vi "App - analyze RUS V6.vi"() -> ()   [LabVIEW 2018] (continued)
              tunnel: w1145 -> [w1161]
              tunnel: w1144 -> [w1159]
              frame #0 {
                n513 = call "cursor window logic V2.vi"("CursIdx"=w1151, "cursor window action"=cursor_window_action."cursor moves", "cursor window in"=w1152) -> ("cursor window out"=w1149:refnum<vi>)  [unwired: 7 in, 1 out]
                n514 = call "single fit V5.vi"("find fit action"=find_peak_action."fragment window moves", "cursor bracket: fragment  ref"=w1149) -> ("single fit parameters out"=w1154:T21, "omega map parameters out"=w1155:T22, "lorentzian out"=w1153:T11)  [unwired: 9 in, 2 out]
                n515 = local write "parameters: center detection"(w1154) -> ()
                n516 = local write "parameters: omega map"(w1155) -> ()
                n517 = local write "lorentzian"(w1153) -> ()
                n518 = Unbundle By Name(w1153) -> ("f (Hz)"=w1157:dbl)
              }
              frame #1 {
                w1160 = enum16{"", "read", "write"}."write"  # action
                w1162 = "update freq/atten"  # t.folder
                n519 = call "replace cursor - plot ref.vi"("action"=w1160, "cursor index"=9, "new X"=w1159, "Plot ref in"=w1161) -> ()  [unwired: 5 in, 3 out]
                n520 = Generate User Event(user event=w1163, event data cluster=w1162) -> ()  [unwired: 2 in, 2 out]
              }
            }
          }
          frame 3 {
            # "blue cursor"
            # "cusor 0 in \"complex plane\", \"geometry \" and l\"inear map \" is tied to cursor in \"fragment\" window"
            n521 = Unbundle By Name(w1166) -> ("normalized z"=w1193:cdb[], "omega in window"=w1192:dbl[], "inverse"=w1169:cdb[], "linear"=w1170:cdb[], "omega around"=w1171:dbl[])
            n522 = call "replace cursor - plot ref.vi"("action"=enum16{"", "read", "write"}."read", "cursor index"=w1189, "Plot ref in"=w1165) -> ("read X"=w1190:dbl)  [unwired: 6 in, 2 out]
            n523 = Threshold 1D Array(2:w1190, 3:w1192) -> (0:w1183:dbl)  [unwired: 1 in]
            n524 = Threshold 1D Array(2:w1190, 3:w1171) -> (0:w1173:dbl)  [unwired: 1 in]
            n525 = Index Array(array=w1193, index=w1183) -> (element=w1188:cdb)
            n526 = Index Array(array=w1170, index=w1173) -> (element=w1175:cdb)
            n527 = Index Array(array=w1171, index=w1173) -> (element=w1172:dbl)
            n528 = Index Array(array=w1169, index=w1173) -> (element=w1182:cdb)
            n529 = Complex To Re/Im(x + iy=w1175) -> (x=w1174:dbl)  [unwired: 1 out]
            n530 = Complex To Re/Im(x + iy=w1182) -> (x=w1179:dbl, y=w1178:dbl)
            n531 = control-ref of="Plot: linear map"() -> (w1168:refnum<vi>)
            n532 = Complex To Re/Im(x + iy=w1188) -> (x=w1187:dbl, y=w1186:dbl)
            n533 = control-ref of="Plot: geometry"() -> (w1167:refnum<vi>)
            n534 = call "replace cursor - plot ref.vi"("action"=enum16{"", "read", "write"}."write" ("Enum"), "cursor index"=0, "new  Y"=w1186, "new X"=w1187, "Plot ref in"=w1164) -> ()  [unwired: 4 in, 3 out]
            n535 = call "replace cursor - plot ref.vi"("action"=enum16{"", "read", "write"}."write" ("Enum"), "cursor index"=0, "new  Y"=w1174, "new X"=w1172, "Plot ref in"=w1168) -> ()  [unwired: 4 in, 3 out]
            n536 = call "replace cursor - plot ref.vi"("action"=enum16{"", "read", "write"}."write" ("Enum"), "cursor index"=0, "new  Y"=w1178, "new X"=w1179, "Plot ref in"=w1167) -> ()  [unwired: 4 in, 3 out]
          }
        }
      }
      event "Plot: Time": Cursor Release {
        w1200 = enum16{"hide", "show x", "show y", "show (x,y)"}."hide"  # label
        w1201 = enum16{"", "read", "write"}."write"  # action
        w1202 = "same"  # next temperature
        n537 = event-data() -> ("CursIdx"=w1198:i32)  [unwired: 1 in]
        n538 = call "replace cursor - plot ref.vi"("label"=w1200, "action"=w1201, "cursor index"=w1198, "Plot ref in"=w1199) -> ()  [unwired: 5 in, 3 out]
        n539 = Generate User Event(user event=w1203, event data cluster=w1202) -> ()  [unwired: 2 in, 2 out]
        n540 = call "slide controller.vi"("slide action"=slide_action."stop slide", "slide control"=w1195) -> ()  [unwired: 6 in, 4 out]
        n541 = call "follow the peak controller.vi"("action"=follow_the_peak_action."make dirty", "follow the peak ref"=w1197) -> ()  [unwired: 8 in, 2 out]
      }
      event Key Down {
        n542 = event-data() -> ("Type"=w1208:T20, "Char"=w1223:i16, "VKey"=w1212:T19)  [unwired: 1 in]
        "Char" <- w1223
        "VKey" <- w1212
        "Type" <- w1208
        n543 = case shown="\"ASCII\", Default" w1212 {
          selector: w1212 -> [_ _ _ _ _ _ _ _ _ _ _ _ w1395 _ _ _ _ _ _ _ _ _ _ _ _ _ _ _ _ _ _ _ _ _ _ _ _ _ _ _ _ _ _ _ _ _ _ _ _ _]
          tunnel: w1223 -> [w1242 _ _ _ _ _ _ _ _ _ _ _ _ _ _ _ _ _ _ _ _ _ _ _ _ _ _ _ _ _ _ _ _ _ _ _ _ _ _ _ _ _ _ _ _ _ _ _ _ _]
          tunnel: w1222 -> [w1241 _ _ _ _ _ _ _ _ _ _ _ _ _ _ _ _ _ _ _ _ _ _ _ _ _ _ _ _ _ _ _ _ _ _ _ _ _ _ _ _ _ _ _ _ _ _ _ _ _]
          tunnel: w1221 -> [w1240 _ _ _ _ _ _ _ _ _ _ _ _ _ _ _ _ _ _ _ _ _ _ _ _ _ _ _ _ _ _ _ _ _ _ _ _ _ _ _ _ _ _ _ _ _ _ _ _ _]
          tunnel: w1220 -> [w1239 _ _ _ _ _ _ _ _ _ _ _ _ _ _ _ _ _ _ _ _ _ _ _ _ _ _ _ _ _ _ _ _ _ _ _ _ _ _ _ _ _ _ _ _ _ _ _ _ _]
          tunnel: w1219 -> [w1238 _ _ _ _ _ _ _ _ _ _ _ _ _ _ _ _ _ _ _ _ _ _ _ _ _ _ _ _ _ _ _ _ _ _ _ _ _ _ _ _ _ _ _ _ _ _ _ _ _]
          tunnel: w1218 -> [w1237 _ _ _ _ _ _ _ _ _ _ _ w1390 _ _ _ _ _ _ _ _ _ _ _ _ _ _ _ _ _ _ _ _ _ _ _ _ _ _ _ _ _ _ _ _ _ _ _ _ _]
          tunnel: w1217 -> [w1236 _ _ _ _ _ _ _ _ _ _ _ _ _ _ _ _ _ _ _ _ _ _ _ _ _ _ _ _ _ _ _ _ _ _ _ _ _ _ _ _ _ _ _ _ _ _ _ _ _]
          tunnel: w1216 -> [w1235 _ _ _ _ _ _ _ _ _ _ _ _ _ _ _ _ _ _ _ _ _ _ _ _ _ _ _ _ _ _ _ _ _ _ _ _ _ _ _ _ _ _ _ _ _ _ _ _ _]
          tunnel: w1215 -> [w1234 _ _ _ _ _ _ _ _ _ _ _ _ _ _ _ _ _ _ _ _ _ _ _ _ _ _ _ _ _ _ _ _ _ _ _ _ _ _ _ _ _ _ _ _ _ _ _ _ _]
          tunnel: w1214 -> [w1233 _ _ _ _ _ _ _ _ _ _ _ w1391 _ _ _ _ _ _ _ _ _ _ _ _ _ _ _ _ _ _ _ _ _ _ _ _ _ _ _ _ _ _ _ _ _ _ _ _ _]
          tunnel: w1213 -> [w1232 _ _ _ _ _ _ _ _ _ _ _ w1394 _ _ _ _ _ _ _ _ _ _ _ _ _ _ _ _ _ _ _ _ _ _ _ _ _ _ _ _ _ _ _ _ _ _ _ _ _]
          tunnel: w1211 -> [w1230 _ _ _ _ _ _ _ _ _ _ _ w1392 _ _ _ _ _ _ _ _ _ _ _ _ _ _ _ _ _ _ _ _ _ _ _ _ _ _ _ _ _ _ _ _ _ _ _ _ _]
          tunnel: w1210 -> [w1231 _ w1383 _ _ _ _ _ _ _ _ _ _ _ _ _ _ _ _ _ _ _ _ _ _ _ _ _ _ _ _ _ _ _ _ _ _ _ _ _ _ _ _ _ _ _ _ _ _ _]
          tunnel: w1209 -> [_ _ w1384 _ _ _ _ _ _ _ _ _ _ _ _ _ _ _ _ _ _ _ _ _ _ _ _ _ _ _ _ _ _ _ _ _ _ _ _ _ _ _ _ _ _ _ _ _ _ _]
          tunnel: w1208 -> [_ _ _ _ _ _ _ _ _ _ _ _ _ _ _ _ _ _ _ _ _ _ _ _ _ _ _ _ _ _ _ _ _ _ _ _ _ _ _ _ _ _ _ _ _ _ _ _ _ _]
          tunnel: w1207 -> [w1227 _ _ _ _ _ _ _ _ _ _ _ _ _ _ _ _ _ _ _ _ _ _ _ _ _ _ _ _ _ _ _ _ _ _ _ _ _ _ _ _ _ _ _ _ _ _ _ _ _]
          tunnel: w1206 -> [w1226 _ _ _ _ _ _ _ _ _ _ _ _ _ _ _ _ _ _ _ _ _ _ _ _ _ _ _ _ _ _ _ _ _ _ _ _ _ _ _ _ _ _ _ _ _ _ _ _ _]
          tunnel: w1205 -> [w1225 _ _ _ _ _ _ _ _ _ _ _ _ _ _ _ _ _ _ _ _ _ _ _ _ _ _ _ _ _ _ _ _ _ _ _ _ _ _ _ _ _ _ _ _ _ _ _ _ _]
          tunnel: w1204 -> [w1224 _ w1380 _ _ _ _ _ _ _ _ _ _ _ _ _ _ _ _ _ _ _ _ _ _ _ _ _ _ _ _ _ _ _ _ _ _ _ _ _ _ _ _ _ _ _ _ _ _ _]
          frame "ASCII", Default {
            # "[  - next temperature -- Down\n]  - next temperature -- Up\n\" \" - recalculate , stop sliding\n>  - start slide Up\n< -  start slide Down\n\netc..."
            n544 = case shown="111" w1242 {
              tunnel: w1241 -> [_ w1254 w1258 _ _ _ _ w1278 w1284 _ _ _ _ _ _ _ _ _ _ _ _ _ _ _ _ _ _ _ _ _ _ _ _]
              tunnel: TRUE -> [_ _ _ _ _ _ _ _ _ _ _ _ _ _ _ _ _ _ _ _ _ _ _ _ _ _ _ _ _ _ _ w1375 _]
              tunnel: w1239 -> [_ _ _ _ _ _ _ _ _ _ _ _ _ _ _ _ _ _ _ _ _ _ _ _ _ _ _ _ _ _ _ _ _]
              tunnel: FALSE -> [_ _ _ _ _ _ _ _ _ _ _ _ _ _ _ _ _ _ _ _ _ _ _ _ _ _ _ _ _ _ _ w1376 _]
              tunnel: w1240 -> [_ _ _ _ _ _ _ _ _ _ _ _ _ _ _ _ _ _ _ _ w1328 _ w1342 _ _ _ _ _ _ _ _ _ _]
              tunnel: w1238 -> [_ _ _ _ _ _ _ _ _ _ _ _ _ _ _ _ _ _ _ _ _ w1340 _ _ _ _ _ _ _ _ _ _ _]
              tunnel: w1237 -> [_ _ _ w1263 _ _ _ _ _ _ _ _ _ _ _ _ _ _ _ _ _ _ _ _ _ _ _ _ _ _ _ w1379 _]
              tunnel: w1236 -> [w1247 _ _ w1260 w1264 w1267 w1271 _ _ _ _ _ _ _ w1305 _ _ _ w1313 _ w1329 _ _ w1348 w1359 w1360 w1362 _ _ _ w1372 _ _]
              tunnel: w1235 -> [_ _ _ _ _ _ _ _ _ _ _ _ _ _ _ _ _ _ _ _ _ _ _ _ _ _ _ _ _ _ _ _ _]
              tunnel: w1234 -> [_ _ _ _ _ _ _ _ _ _ _ _ _ w1302 _ _ _ _ _ _ _ _ _ _ _ _ _ _ _ _ _ _ _]
              tunnel: w1233 -> [_ _ _ _ _ _ _ _ _ _ _ _ w1293 _ _ _ _ _ _ _ _ _ _ _ _ _ _ _ _ _ _ _ _]
              tunnel: w1232 -> [w1249 _ _ _ _ _ _ _ _ _ w1287 w1289 _ _ _ _ _ _ _ w1315 _ _ _ _ _ _ _ w1366 w1368 w1370 _ _ _]
              tunnel: w1231 -> [_ _ _ _ _ _ _ _ _ _ _ _ _ _ _ _ _ _ _ w1318 _ _ _ _ _ _ _ _ _ _ _ _ _]
              tunnel: w1230 -> [_ _ _ _ _ _ _ _ _ w1285 _ _ _ _ _ _ _ _ _ w1319 _ _ _ _ _ _ _ _ _ _ _ _ _]
              tunnel: w1227 -> [_ _ _ _ _ _ _ _ _ _ _ _ _ _ _ _ _ _ _ _ _ _ _ _ _ _ _ _ _ _ _ _ _]
              tunnel: w1226 -> [w1246 _ _ _ _ _ _ _ _ _ _ _ _ _ _ w1307 w1310 _ _ _ _ _ _ _ _ _ _ _ _ _ _ _ _]
              tunnel: w1225 -> [w1243 w1252 w1255 _ _ _ _ w1273 w1281 _ _ _ _ _ _ _ _ _ _ _ _ _ _ _ _ _ _ _ _ _ _ _ _]
              tunnel: w1224 -> [_ _ _ _ _ _ _ _ _ _ _ _ _ _ w1303 _ _ _ _ _ _ _ _ w1343 w1356 _ _ _ _ _ _ _ _]
              frame 32 {
                w1248 = "update delta freq"  # t.folder
                # "stop slide and/or recalculate"
                # "\"<space>\""
                # "recalculate"
                n545 = Generate User Event(user event=w1249, event data cluster="calc:peak" ("event data")) -> ()  [unwired: 2 in, 2 out]
                n546 = call "follow the peak controller.vi"("action"=follow_the_peak_action."make dirty", "follow the peak ref"=w1246) -> ()  [unwired: 8 in, 2 out]
                n547 = call "slide controller.vi"("slide action"=slide_action."stop slide", "slide control"=w1243) -> ()  [unwired: 6 in, 4 out]
                n548 = Generate User Event(user event=w1247, event data cluster=w1248) -> ()  [unwired: 2 in, 2 out]
              }
              frame 44 {
                w1253 = "next"  # event data
                # "slide down"
                # "\" <\""
                n549 = Generate User Event(user event=w1254, event data cluster=w1253) -> ()  [unwired: 2 in, 2 out]
                n550 = call "slide controller.vi"("slide action"=slide_action."slide DOWN", "slide control"=w1252) -> ()  [unwired: 6 in, 4 out]
              }
              frame 46 {
                w1257 = "next"  # event data
                # "slide up"
                # ">"
                n551 = Generate User Event(user event=w1258, event data cluster=w1257) -> ()  [unwired: 2 in, 2 out]
                n552 = call "slide controller.vi"("slide action"=slide_action."slide UP", "slide control"=w1255) -> ()  [unwired: 6 in, 4 out]
              }
              frame 47 {
                w1261 = "update delta freq"  # t.folder
                (unwired) FALSE ("event data")
                # "\"/\""
                n553 = Generate User Event(user event=w1263, event data cluster="scale:frequency window" ("event data")) -> (error out=w1259:errorcluster)  [unwired: 2 in, 1 out]
                n554 = Generate User Event(user event=w1260, event data cluster=w1261, error in=w1259) -> ()  [unwired: 1 in, 2 out]
              }
              frame 59 {
                w1265 = "next peak"  # event data
                n555 = Generate User Event(user event=w1264, event data cluster=w1265) -> ()  [unwired: 2 in, 2 out]
              }
              frame 39 {
                n556 = for {
                  tunnel: w1267 -> [w1270]
                  tunnel: string[] ["write freq file", "increment peak index", "clear freq points", "follow the peak -- init", "set time to left", "read freq file"] -> [w1268] mode=indexing
                  n557 = Wait (ms)(milliseconds to wait=u32 1000) -> ()  [unwired: 1 out]
                  n558 = Generate User Event(user event=w1270, event data cluster=w1268) -> ()  [unwired: 2 in, 2 out]
                  "script event" <- w1268
                }
              }
              frame 58 {
                w1272 = "increment peak index"  # event data
                n559 = Generate User Event(user event=w1271, event data cluster=w1272) -> ()  [unwired: 2 in, 2 out]
              }
              frame 60 {
                w1277 = "next"  # next temperature
                # "next DOWN"
                # "shift <"
                # "send \"next temperature"
                # "next temperature  -- Down"
                n560 = Generate User Event(user event=w1278, event data cluster=w1277) -> ()  [unwired: 2 in, 2 out]
                n561 = call "slide controller.vi"("slide action"=slide_action."slide DOWN", "slide control"=w1273) -> ("slide control OUT"=w1274:refnum<vi>)  [unwired: 6 in, 3 out]
                n562 = call "slide controller.vi"("slide action"=slide_action."stop slide", "slide control"=w1274) -> ()  [unwired: 6 in, 4 out]
              }
              frame 62 {
                w1283 = "next"  # next temperature
                (unwired) TRUE
                (unwired) -1
                (unwired) 1
                # "next UP"
                # "shift >"
                # "Up"
                # "send next temperature"
                n563 = Generate User Event(user event=w1284, event data cluster=w1283) -> ()  [unwired: 2 in, 2 out]
                n564 = call "slide controller.vi"("slide action"=slide_action."slide UP", "slide control"=w1281) -> ("slide control OUT"=w1280:refnum<vi>)  [unwired: 6 in, 3 out]
                n565 = call "slide controller.vi"("slide action"=slide_action."stop slide", "slide control"=w1280) -> ()  [unwired: 6 in, 4 out]
              }
              frame 63 {
                n566 = call "cursor window logic V2.vi"("cursor window action"=cursor_window_action."zoom X", "cursor window in"=w1285) -> ()  [unwired: 8 in, 2 out]
              }
              frame 92 {
                w1288 = "jump to a PID peak"  # calculate
                # "\"\\\""
                n567 = Generate User Event(user event=w1287, event data cluster=w1288) -> ()  [unwired: 2 in, 2 out]
              }
              frame 43 {
                w1290 = "overwrite peak PID"  # calculate
                # "\"\\\""
                n568 = Generate User Event(user event=w1289, event data cluster=w1290) -> ()  [unwired: 2 in, 2 out]
              }
              frame 97 {
                # "\"a\""
                # "all plot autoscale"
                # "\"a\""
                n569 = local read "all:max omega"() -> (w1299:dbl)
                n570 = local read "all:min omega"() -> (w1298:dbl)
                n571 = Add(x=w1299, y=w1298) -> (x+y=w1300:dbl)
                n572 = Subtract(x=w1299, y=w1298) -> (x-y=w1297:dbl)
                n573 = Divide(x=w1300, y=2.0) -> (x/y=w1294:dbl)
                n574 = Divide(x=w1297, y=1.5) -> (x/y=w1291:dbl)
                n575 = property on="Plot: All" class="XYGraph (strict)"("XScale.Maximum"=w1299, "XScale.Minimum"=w1298) -> ()  [unwired: 2 in, 2 out]
                n576 = call "cursor window logic V2.vi"("cursor window action"=cursor_window_action."change cen&win", "window"=w1291, "center"=w1294, "cursor window in"=w1293) -> ()  [unwired: 6 in, 2 out]
              }
              frame 99 {
                (unwired) 0.0 ("event data")
                # "show cursors"
                # "\"c\""
                n577 = Generate User Event(user event=w1302, event data cluster="cursors:check all" ("event data")) -> ()  [unwired: 2 in, 2 out]
              }
              frame 101 {
                w1306 = "clear freq points"  # t.folder
                # "erase freq points \n\nshortcut \"e\""
                n578 = Generate User Event(user event=w1305, event data cluster=w1306) -> ()  [unwired: 2 in, 2 out]
                n579 = call "freq file read-write controller.vi"("action"=save-read_action."erase event", "save/read"=w1303) -> ()  [unwired: 7 in, 3 out]
              }
              frame 102 {
                # "\"f\""
                n580 = call "follow the peak controller.vi"("action"=follow_the_peak_action."toggle omega", "follow the peak ref"=w1307) -> ()  [unwired: 8 in, 2 out]
              }
              frame 103 {
                n581 = call "follow the peak controller.vi"("action"=follow_the_peak_action."toggle gamma", "follow the peak ref"=w1310) -> ()  [unwired: 8 in, 2 out]
              }
              frame 104 {
                # "help  \"h\""
                n582 = local read "help toggle"() -> (w1312:bool)
                n583 = Not(x=w1312) -> (.not. x?=w1311:bool)
                n584 = local write "help toggle"(w1311) -> ()
                n585 = Control Help Window(1:w1311) -> ()  [unwired: 1 in]
              }
              frame 106 {
                # "j"
                n586 = Generate User Event(user event=w1313, event data cluster="set time to left" ("event data")) -> ()  [unwired: 2 in, 2 out]
              }
              frame 109 {
                # "\"m\""
                n587 = Unbundle By Name(w1318) -> ("f (Hz)"=w1316:dbl)
                n588 = call "Q - not nan and not zero.vi"("Numeric"=w1316) -> ("Boolean"=w1317:bool)  [unwired: 10 in]
                n589 = case shown="True" w1317 {
                  tunnel: w1319 -> [_ w1322]
                  tunnel: w1316 -> [_ w1321]
                  tunnel: w1315 -> [_ w1320]
                  frame False {
                  }
                  frame True {
                    n590 = flat-sequence {
                      tunnel: w1322 -> [w1325]
                      tunnel: w1321 -> [w1324]
                      tunnel: w1320 -> [w1326]
                      frame #0 {
                        n591 = call "cursor window logic V2.vi"("cursor window action"=cursor_window_action."check", "center"=w1324, "cursor window in"=w1325) -> ()  [unwired: 7 in, 2 out]
                      }
                      frame #1 {
                        w1327 = "calc:new cursor bracket"  # event data
                        n592 = Generate User Event(user event=w1326, event data cluster=w1327) -> ()  [unwired: 2 in, 2 out]
                      }
                    }
                  }
                }
              }
              frame 111 {
                # "\"o\""
                n593 = flat-sequence {
                  tunnel: w1329 -> [w1332]
                  tunnel: [w1331] -> w1330
                  tunnel: [w1334] -> _
                  tunnel: w1330 -> [w1335]
                  tunnel: w1328 -> [w1336]
                  frame #0 {
                    w1333 = "new temperature folder"  # t.folder
                    n594 = Generate User Event(user event=w1332, event data cluster=w1333) -> (error out=w1331:errorcluster)  [unwired: 2 in, 1 out]
                  }
                  frame #1 {
                    n595 = Generate User Event(user event=w1336, event data cluster="redraw:time", error in=w1335) -> (error out=w1334:errorcluster)  [unwired: 1 in, 1 out]
                  }
                }
              }
              frame 112 {
                # "\"p\""
                n596 = local read "show all pallets (p)"() -> (w1339:bool)
                n597 = Not(x=w1339) -> (.not. x?=w1338:bool)
                n598 = local write "show all pallets (p)"(w1338) -> ()
                n599 = Generate User Event(user event=w1340, event data cluster=w1338) -> ()  [unwired: 2 in, 2 out]
              }
              frame 113 {
                w1341 = "plot filter progress"  # event data
                # "q"
                n600 = Generate User Event(user event=w1342, event data cluster=w1341) -> ()  [unwired: 2 in, 2 out]
              }
              frame 114 {
                w1350 = "update delta freq"  # t.folder
                w1351 = "read freq file"  # t.folder
                # "make something to protect  from overwriting a file"
                # "\"r\""
                n601 = case shown="True" FALSE {
                  tunnel: w1348 -> [w1352 w1354]
                  tunnel: [w1352 w1353] -> w1347
                  frame False {
                  }
                  frame True {
                    w1355 = "clear freq points"  # t.folder
                    n602 = Generate User Event(user event=w1354, event data cluster=w1355) -> (user event out=w1353:refnum<user-event>)  [unwired: 2 in, 1 out]
                  }
                }
                n603 = call "freq file read-write controller.vi"("action"=save-read_action."read event", "save/read"=w1343) -> ()  [unwired: 7 in, 3 out]
                n604 = Generate User Event(user event=w1347, event data cluster=w1351) -> (user event out=w1349:refnum<user-event>, error out=w1346:errorcluster)  [unwired: 2 in]
                n605 = Generate User Event(user event=w1349, event data cluster=w1350, error in=w1346) -> ()  [unwired: 1 in, 2 out]
              }
              frame 115 {
                w1358 = "write freq file"  # t.folder
                # "\"s\""
                n606 = call "freq file read-write controller.vi"("action"=save-read_action."save event", "save/read"=w1356) -> ()  [unwired: 7 in, 3 out]
                n607 = Generate User Event(user event=w1359, event data cluster=w1358) -> ()  [unwired: 2 in, 2 out]
              }
              frame 116 {
                w1361 = "lookup read from list"  # t.folder
                # "\"t\""
                n608 = Generate User Event(user event=w1360, event data cluster=w1361) -> ()  [unwired: 2 in, 2 out]
              }
              frame 117 {
                w1363 = "latest temperature"  # t.folder
                n609 = disable-structure shown="Disabled" {
                  disable-tunnel: w1362 -> [w1364 _]
                  frame Disabled {
                    w1365 = "append frequency PID file"  # t.folder
                    # "\"u\""
                    n610 = Generate User Event(user event=w1364, event data cluster=w1365) -> ()  [unwired: 2 in, 2 out]
                  }
                  frame Enabled {
                  }
                }
                n611 = Generate User Event(user event=w1362, event data cluster=w1363) -> ()  [unwired: 2 in, 2 out]
              }
              frame 118 {
                w1367 = "scan for existing peaks"  # calculate
                # "\"v\""
                n612 = Generate User Event(user event=w1366, event data cluster=w1367) -> ()  [unwired: 2 in, 2 out]
              }
              frame 119 {
                w1369 = "save cursor window"  # calc
                # "w"
                n613 = Generate User Event(user event=w1368, event data cluster=w1369) -> ()  [unwired: 2 in, 2 out]
              }
              frame 120 {
                # "\"x\""
                n614 = Generate User Event(user event=w1370, event data cluster="calc: scan" ("t.folder")) -> ()  [unwired: 2 in, 2 out]
              }
              frame 121 {
                # "\"y\""
                n615 = Generate User Event(user event=w1372, event data cluster="write RPR line" ("t.folder")) -> ()  [unwired: 2 in, 2 out]
              }
              frame 122 {
                # "zoom in/out c.plane plot"
                # "\"z\""
                n616 = local read "c.plane scale"() -> (w1377:bool)
                n617 = Select(t=w1376, s=w1377, f=w1375) -> (s? t:f=w1374:bool)
                n618 = local write "c.plane scale"(w1374) -> ()
                n619 = Generate User Event(user event=w1379, event data cluster="scale:c.plane plot zoom" ("event data")) -> ()  [unwired: 2 in, 2 out]
              }
              frame Default {
              }
            }
          }
          frame "Enter" {
          }
          frame "Return" {
            n620 = Unbundle By Name(w1383) -> ("f (Hz)"=w1382:dbl)
            n621 = call "Q - not nan and not zero.vi"("Numeric"=w1382) -> ("Boolean"=w1381:bool)  [unwired: 10 in]
            n622 = Compound Arithmetic op=AND(w1381, w1384) -> (w1385:bool)
            n623 = case shown="True" w1385 {
              tunnel: w1382 -> [_ w1386]
              tunnel: w1380 -> [_ w1387]
              frame False {
              }
              frame True {
                n624 = call "freq file read-write controller.vi"("action"=save-read_action."set save file", "Numeric"=w1386, "save/read"=w1387) -> ()  [unwired: 6 in, 3 out]
              }
            }
          }
          frame "Shift" {
          }
          frame "Ctrl" {
          }
          frame "Alt" {
          }
          frame "Cmd" {
          }
          frame "Opt" {
          }
          frame "Caps" {
          }
          frame "NumLock" {
          }
          frame "Clear" {
          }
          frame "Break" {
          }
          frame "Up".."Right", "PageUp", "PageDown" {
            n625 = flat-sequence {
              tunnel: w1393 -> [w1398]
              tunnel: w1395 -> [w1400]
              tunnel: "Up/Down/Left/Right target" -> [w1399]
              tunnel: w1394 -> [w1415]
              tunnel: "Up/Down/Left/Right target" -> [w1414]
              tunnel: w1390 -> [w1413]
              frame #0 {
                n626 = case shown="\"Up\"" w1400 {
                  tunnel: w1399 -> [_ _ _ _ _ _]
                  tunnel: w1398 -> [w1401 w1403 w1405 w1407 w1409 w1412]
                  frame "Right", Default {
                    n627 = call "cursor window logic V2.vi"("cursor window action"=cursor_window_action."move right", "cursor window in"=w1401) -> ()  [unwired: 8 in, 2 out]
                  }
                  frame "Left" {
                    n628 = call "cursor window logic V2.vi"("cursor window action"=cursor_window_action."move left", "cursor window in"=w1403) -> ()  [unwired: 8 in, 2 out]
                  }
                  frame "PageUp" {
                    n629 = call "cursor window logic V2.vi"("cursor window action"=cursor_window_action."skew up", "cursor window in"=w1405) -> ()  [unwired: 8 in, 2 out]
                  }
                  frame "PageDown" {
                    n630 = call "cursor window logic V2.vi"("cursor window action"=cursor_window_action."skew down", "cursor window in"=w1407) -> ()  [unwired: 8 in, 2 out]
                  }
                  frame "Up" {
                    n631 = call "cursor window logic V2.vi"("cursor window action"=cursor_window_action."broaden", "cursor window in"=w1409) -> ()  [unwired: 8 in, 2 out]
                  }
                  frame "Down" {
                    n632 = call "cursor window logic V2.vi"("cursor window action"=cursor_window_action."shrink", "cursor window in"=w1412) -> ()  [unwired: 8 in, 2 out]
                  }
                }
              }
              frame #1 {
                n633 = case shown="\"window cursor\"" w1414 {
                  tunnel: w1415 -> [_ w1418]
                  tunnel: w1413 -> [w1416 _]
                  frame "zoom cursor", Default {
                    w1417 = "rescale All from Zoom cursor"  # event data
                    n634 = Generate User Event(user event=w1416, event data cluster=w1417) -> ()  [unwired: 2 in, 2 out]
                  }
                  frame "window cursor" {
                    w1419 = "calc:new cursor bracket"  # event data
                    n635 = Generate User Event(user event=w1418, event data cluster=w1419) -> ()  [unwired: 2 in, 2 out]
                  }
                }
              }
            }
            n636 = case shown="\"window cursor\"" "Up/Down/Left/Right target" {
              tunnel: [w1396 w1397] -> w1393
              tunnel: w1392 -> [_ w1397]
              tunnel: w1391 -> [w1396 _]
              frame "zoom cursor", Default {
              }
              frame "window cursor" {
              }
            }
          }
          frame "Insert" {
          }
          frame "Delete" {
          }
          frame "Home" {
          }
          frame "End" {
          }
          frame "Escape" {
            n637 = control-ref of="Up/Down/Left/Right target"() -> (w1423:refnum<vi>)
            n638 = property class="Enum (strict)"(reference=w1423) -> (reference out=w1422:refnum<vi>, "Value"=w1420:enum16{"zoom cursor", "window cursor"})  [unwired: 1 in, 1 out]
            n639 = case shown="\"zoom cursor\", Default" w1420 {
              tunnel: [enum16{"zoom cursor", "window cursor"}."window cursor" ("Value") enum16{"zoom cursor", "window cursor"}."zoom cursor" ("Value")] -> w1421
              frame "zoom cursor", Default {
              }
              frame "window cursor" {
              }
            }
            n640 = property class="Enum (strict)"(reference=w1422, "Value"=w1421) -> ()  [unwired: 1 in, 2 out]
          }
          frame "Help" {
          }
          frame "Pause" {
          }
          frame "ScrollLock" {
          }
          frame "F1" {
          }
          frame "F2" {
          }
          frame "F3" {
          }
          frame "F4" {
          }
          frame "F5" {
          }
          frame "F6" {
          }
          frame "F7" {
          }
          frame "F8" {
          }
          frame "F9" {
          }
          frame "F10" {
          }
          frame "F11" {
          }
          frame "F12" {
          }
          frame "F13" {
          }
          frame "F14" {
          }
          frame "F15" {
          }
          frame "F16" {
          }
          frame "F17" {
          }
          frame "F18" {
          }
          frame "F19" {
          }
          frame "F20" {
          }
          frame "F21" {
          }
          frame "F22" {
          }
          frame "F23" {
          }
          frame "F24" {
          }
          frame "Play" {
          }
          frame "VolumeUp" {
          }
          frame "VolumeDown" {
          }
          frame "Mute" {
          }
          frame "Two Byte Char" {
          }
        }
      }
      event "Plot: complex plane": Cursor Move {
        n641 = event-data() -> ("CursIdx"=w1433:i32)  [unwired: 1 in]
        n642 = flat-sequence {
          tunnel: w1433 -> [w1443]
          tunnel: [w1440] -> w1431
          tunnel: w1430 -> [w1438]
          tunnel: w1429 -> [w1437]
          tunnel: w1428 -> [w1436]
          tunnel: w1427 -> [w1435]
          tunnel: w1426 -> [w1434]
          tunnel: w1432 -> [w1471]
          tunnel: w1431 -> [w1470]
          frame #0 {
            n643 = case shown="2" w1443 {
              selector: w1443 -> [_ w1457 w1465]
              tunnel: w1436 -> [w1444 _ _]
              tunnel: [w1447 w1449 w1459] -> w1442
              tunnel: w1438 -> [w1447 _ _]
              tunnel: [FALSE TRUE TRUE] -> w1440
              tunnel: [w1445 w1448 w1460] -> w1441
              tunnel: w1437 -> [w1445 _ _]
              tunnel: w1434 -> [_ _ _]
              tunnel: [w1444 w1450 w1461] -> w1439
              tunnel: w1435 -> [_ w1453 w1464]
              frame 0, Default {
              }
              frame 1 {
                # "replace z(inf)  -- keeping z(center) the same"
                n644 = call "replace cursor - plot ref.vi"("action"=enum16{"", "read", "write"}."read" ("Enum"), "cursor index"=w1457, "Plot ref in"=w1453) -> ("read Y"=w1455:dbl, "read X"=w1456:dbl)  [unwired: 6 in, 1 out]
                n645 = Re/Im To Complex(1:w1455, 2:w1456) -> (0:w1451:cdb)
                n646 = call "single fit V5.vi"("find fit action"=find_peak_action."move z(inf)", "input"=w1451) -> ("single fit parameters out"=w1450:T21, "omega map parameters out"=w1448:T22, "lorentzian out"=w1449:T11)  [unwired: 9 in, 2 out]
              }
              frame 2 {
                # "replace z(center) -- keepin z(inf) the same"
                n647 = call "replace cursor - plot ref.vi"("action"=enum16{"", "read", "write"}."read" ("Enum"), "cursor index"=w1465, "Plot ref in"=w1464) -> ("read Y"=w1467:dbl, "read X"=w1468:dbl)  [unwired: 6 in, 1 out]
                n648 = Re/Im To Complex(1:w1467, 2:w1468) -> (0:w1462:cdb)
                n649 = call "single fit V5.vi"("find fit action"=find_peak_action."move z(center)", "input"=w1462) -> ("single fit parameters out"=w1461:T21, "omega map parameters out"=w1460:T22, "lorentzian out"=w1459:T11)  [unwired: 9 in, 2 out]
              }
            }
            n650 = local write "parameters: center detection"(w1439) -> ()
            n651 = local write "lorentzian"(w1442) -> ()
            n652 = local write "parameters: omega map"(w1441) -> ()
          }
          frame #1 {
            n653 = case shown="True" w1470 {
              tunnel: w1471 -> [_ w1473]
              frame False {
              }
              frame True {
                w1472 = "update freq/atten"  # t.folder
                n654 = Generate User Event(user event=w1473, event data cluster=w1472) -> ()  [unwired: 2 in, 2 out]
              }
            }
          }
        }
      }
      event User Event {
        # "load file for the current temperature"
        n655 = event-data() -> ("next temperature"=w1484:string)  [unwired: 1 in]
        n656 = local read "time (min)"() -> (w1479:dbl)
        n657 = call "PCRE-exact match.vi"("regular expression"="(next|same)", "input string"=w1484) -> ("exact match"=w1482:bool)  [unwired: 7 in, 2 out]
        n658 = call "slide controller.vi"("slide action"=slide_action."check", "slide control"=w1475) -> ("slide control OUT"=w1474:T4)  [unwired: 6 in, 3 out]
        n659 = Unbundle By Name(w1474) -> ("direction"=w1477:bool)
        n660 = And(x=w1482, y=w1481) -> (x .and. y?=w1480:bool)
        n661 = local read "time points"() -> (w1478:dbl[])
        n662 = case shown="True" w1480 {
          tunnel: w1486 -> [_ w1493]
          tunnel: w1484 -> [_ w1494]
          tunnel: w1485 -> [_ w1492]
          tunnel: w1479 -> [_ w1491]
          tunnel: w1478 -> [_ w1490]
          tunnel: w1477 -> [_ w1489]
          tunnel: w1475 -> [_ w1487]
          frame False {
          }
          frame True {
            n663 = case shown="\"next\"" w1494 {
              tunnel: w1491 -> [_ w1510]
              tunnel: w1492 -> [_ w1509]
              tunnel: w1490 -> [_ w1503]
              tunnel: w1489 -> [_ w1507]
              tunnel: [TRUE w1504] -> w1488
              frame "same", Default {
                # "load current temperature file"
              }
              frame "next" {
                # "calculate next temperature"
                n664 = Threshold 1D Array(2:w1510, 3:w1503) -> (0:w1501:dbl)  [unwired: 1 in]
                n665 = Array Size(array=w1503) -> (size(s)=w1505:i32)
                n666 = Select(t=1, s=w1507, f=-1) -> (s? t:f=w1511:i32)
                n667 = Add(x=w1501, y=w1511) -> (x+y=w1506:dbl)
                n668 = case shown="True" FALSE {
                  tunnel: w1509 -> [_ w1544]
                  tunnel: w1506 -> [w1517 w1543]
                  tunnel: w1505 -> [w1516 _]
                  tunnel: [w1519 TRUE] -> w1504
                  tunnel: w1503 -> [_ w1541]
                  tunnel: [w1515 w1539] -> w1502
                  tunnel: w1501 -> [w1514 _]
                  frame False {
                    w1518 = FALSE  # periodic?
                    n669 = Less?(x=w1517, y=0.0) -> (x < y?=w1520:bool)
                    n670 = Greater Or Equal?(x=w1517, y=w1516) -> (x >= y?=w1521:bool)
                    n671 = Or(x=w1521, y=w1520) -> (x .or. y?=w1522:bool)
                    n672 = case shown="True" w1522 {
                      tunnel: [TRUE w1530] -> w1519
                      tunnel: w1518 -> [_ w1531]
                      tunnel: w1517 -> [w1524 w1529]
                      tunnel: w1516 -> [_ w1528]
                      tunnel: [w1524 w1527] -> w1515
                      tunnel: w1514 -> [_ w1526]
                      frame False {
                      }
                      frame True {
                        n673 = case shown="True" w1531 {
                          tunnel: [FALSE TRUE] -> w1530
                          tunnel: w1529 -> [_ w1536]
                          tunnel: w1528 -> [_ w1535]
                          tunnel: [w1533 w1534] -> w1527
                          tunnel: w1526 -> [w1533 _]
                          frame False {
                          }
                          frame True {
                            n674 = Quotient & Remainder(x=w1536, y=w1535) -> (x-y*floor(x/y)=w1534:dbl)  [unwired: 1 out]
                          }
                        }
                      }
                    }
                  }
                  frame True {
                    n675 = Unbundle By Name(w1544) -> ("left"=w1549:dbl, "right"=w1551:dbl, "window"=w1547:dbl)
                    n676 = Index Array(array=w1541, index=w1543) -> (element=w1542:dbl)
                    n677 = Greater Or Equal?(x=w1542, y=w1551) -> (x >= y?=w1552:bool)
                    n678 = Subtract(x=w1542, y=w1547) -> (x-y=w1550:dbl)
                    n679 = Select(t=w1550, s=w1552, f=w1542) -> (s? t:f=w1545:dbl)
                    n680 = Less Or Equal?(x=w1545, y=w1549) -> (x <= y?=w1548:bool)
                    n681 = Add(x=w1545, y=w1547) -> (x+y=w1546:dbl)
                    n682 = Select(t=w1546, s=w1548, f=w1545) -> (s? t:f=w1540:dbl)
                    n683 = Threshold 1D Array(2:w1540, 3:w1541) -> (0:w1539:dbl)  [unwired: 1 in]
                  }
                }
                n684 = local write "current index"(w1502) -> ()
                n685 = Index Array(array=w1503, index=w1502) -> (element=w1500:dbl)
                n686 = local write "time (min)"(w1500) -> ()
              }
            }
            n687 = case shown="True" w1488 {
              tunnel: w1493 -> [_ w1498]
              tunnel: w1487 -> [w1496 _]
              frame False {
                n688 = call "slide controller.vi"("slide action"=slide_action."start slide", "slide control"=w1496) -> ()  [unwired: 6 in, 4 out]
              }
              frame True {
                n689 = Generate User Event(user event=w1498, event data cluster="new temperature" ("event data")) -> ()  [unwired: 2 in, 2 out]
              }
            }
          }
        }
      }
      event Value Change {
        # "start  temperature slide"
        n690 = event-data() -> ()  [unwired: 1 in, 1 out]
        n691 = case shown="True" w1556 {
          tunnel: w1557 -> [_ w1559]
          frame False {
          }
          frame True {
            w1558 = "next"  # next temperature
            n692 = Generate User Event(user event=w1559, event data cluster=w1558) -> ()  [unwired: 2 in, 2 out]
          }
        }
        n693 = call "slide controller.vi"("slide action"=slide_action."run", "slide control"=w1553) -> ()  [unwired: 6 in, 4 out]
      }
      event Value Change {
        w1564 = "next"  # next temperature
        (unwired) 0.0
        n694 = event-data() -> ()  [unwired: 1 in, 1 out]
        n695 = Generate User Event(user event=w1565, event data cluster=w1564) -> (error out=w1563:errorcluster)  [unwired: 2 in, 1 out]
        n696 = call "slide controller.vi"("slide action"=slide_action."un-next", "slide control"=w1560) -> ()  [unwired: 6 in, 4 out]
      }
      event "Plot: All": Cursor Release {
        n697 = event-data() -> ("CursIdx"=w1574:i32)  [unwired: 1 in]
        n698 = case shown="0..2" w1574 {
          tunnel: w1577 -> [_ w1590]
          tunnel: w1576 -> [_ _]
          tunnel: w1575 -> [_ _]
          tunnel: [w1578 w1585] -> w1571
          tunnel: w1573 -> [w1580 w1592]
          tunnel: w1572 -> [_ w1591]
          tunnel: FALSE ("Boolean") -> [_ _]
          tunnel: TRUE ("Boolean") -> [_ _]
          tunnel: w1568 -> [_ _]
          tunnel: w1567 -> [_ w1584]
          tunnel: w1566 -> [_ w1582]
          frame 3..5, Default {
            w1579 = "rescale All from Zoom cursor"  # event data
            n699 = Generate User Event(user event=w1580, event data cluster=w1579) -> (error out=w1578:errorcluster)  [unwired: 2 in, 1 out]
          }
          frame 0..2 {
            # "select new cursor window"
            # "new cursor"
            n700 = call "follow the peak controller.vi"("action"=follow_the_peak_action."make dirty", "follow the peak ref"=w1584) -> ()  [unwired: 8 in, 2 out]
            n701 = call "slide controller.vi"("slide action"=slide_action."stop slide", "slide control"=w1582) -> ()  [unwired: 6 in, 4 out]
            n702 = Generate User Event(user event=w1590, event data cluster="calc:new cursor bracket" ("event data")) -> (error out=w1587:errorcluster)  [unwired: 2 in, 1 out]
            n703 = Generate User Event(user event=w1592, event data cluster="scale:frequency window" ("event data"), error in=w1587) -> (error out=w1586:errorcluster)  [unwired: 1 in, 1 out]
            n704 = disable-structure shown="Enabled" {
              disable-tunnel: w1591 -> [w1596 _]
              disable-tunnel: w1586 -> [w1594 w1597]
              disable-tunnel: [w1593 w1597] -> w1585
              frame Disabled {
                n705 = Generate User Event(user event=w1596, event data cluster="cursors:check all" ("event data"), error in=w1594) -> (error out=w1593:errorcluster)  [unwired: 1 in, 1 out]
              }
              frame Enabled {
              }
            }
          }
        }
      }
      event "Plot: frequency vs T": Scale Range Change {
        n706 = event-data() -> ("NewRange"=w1598:T42)  [unwired: 1 in]
        n707 = property on="Plot: attenuation vs T" class="XYGraph (strict)"("XScale.Range"=w1598) -> (error out=w1600:errorcluster)  [unwired: 2 in, 1 out]
        n708 = property on="Plot: delta f" class="XYGraph (strict)"(error in=w1600, "XScale.Range"=w1598) -> (error out=w1599:errorcluster)  [unwired: 1 in, 1 out]
      }
      event "c.plane scale": Value Change {
        n709 = event-data() -> ()  [unwired: 1 in, 5 out]
        n710 = Generate User Event(user event=w1602, event data cluster="scale:c.plane plot zoom" ("event data")) -> (error out=w1603:errorcluster)  [unwired: 2 in, 1 out]
      }
      event "show all cursors (c)": Value Change {
        n711 = event-data() -> ()  [unwired: 1 in, 1 out]
        n712 = Generate User Event(user event=w1607, event data cluster="cursors:check all" ("event data")) -> (error out=w1606:errorcluster)  [unwired: 2 in, 1 out]
      }
      event "time (min)": Value Change {
        w1610 = "same"  # t.folder
        n713 = event-data() -> ()  [unwired: 1 in, 1 out]
        n714 = Generate User Event(user event=w1611, event data cluster=w1610) -> (error out=w1609:errorcluster)  [unwired: 2 in, 1 out]
      }
      event "show all pallets (p)": Value Change {
        n715 = event-data() -> ("NewVal"=w1613:bool)  [unwired: 1 in, 1 out]
        n716 = Generate User Event(user event=w1614, event data cluster=w1613) -> (error out=w1612:errorcluster)  [unwired: 2 in, 1 out]
      }
      event User Event {
        w1623 = TRUE ("Allow Multiple Colors")
        n717 = event-data() -> ("colors"=w1616:bool)  [unwired: 1 in]
        n718 = property on="Tab :  Fit controls" class="TabCtl (strict)"("MultColors"=w1623) -> ()  [unwired: 2 in, 2 out]
        n719 = property on="Tab : temperature folder" class="TabCtl (strict)"("MultColors"=w1623) -> ()  [unwired: 2 in, 2 out]
        n720 = property on="Tab : everything" class="TabCtl (strict)"("MultColors"=w1623) -> ()  [unwired: 2 in, 2 out]
        n721 = property on="Tab : everything" class="TabCtl (strict)"() -> ("Colors"=w1622:T43)  [unwired: 2 in, 2 out]
        n722 = property on="Tab : temperature folder" class="TabCtl (strict)"() -> ("Colors"=w1620:T43)  [unwired: 2 in, 2 out]
        n723 = property on="Tab :  Fit controls" class="TabCtl (strict)"() -> ("Colors"=w1621:T43)  [unwired: 2 in, 2 out]
        n724 = case shown="True" w1616 {
          tunnel: w1622 -> [w1629 w1641]
          tunnel: w1621 -> [w1628 w1639]
